vi "SetPersistentConfiguration.vi"(8 "ErrorIn":errorcluster, 9 "DataIn":variant, 11 "ReferenceIn":refnum<class "DemoApplication.lvclass">) -> (0 "ErrorOut":errorcluster, 1 "DataOut":variant, 3 "ReferenceOut":refnum<class "DemoApplication.lvclass">)   [LabVIEW 2021, in "DemoApplication.lvclass"]
uses:
  DemoApplication.lvclass
  C:/Localdata/Projects/TriekselSoft/TriekselsoftApplicationFramework/Source/.Externals/Library_TAF_ApplicationFramework/MasterGUI/MasterGUI.lvclass
  .Externals/Library_TAF_ApplicationFramework/MasterGUI/MasterGUI_MessageData.ctl
  a2d9dd7e-4f73-47a2-b010-087cab1955c7.vi
  7e5dec9a-bf4d-41f7-98bf-8bf962ae9346.vi
  <vilib>/Utility/LVClass/Get LV Class Name.vi
  .Externals/Library_TAF_ApplicationFramework/MasterGUI/MainGUIRepository.vi
  .Externals/Library_TAF_ApplicationFramework/MasterGUI/MasterGUI.lvclass
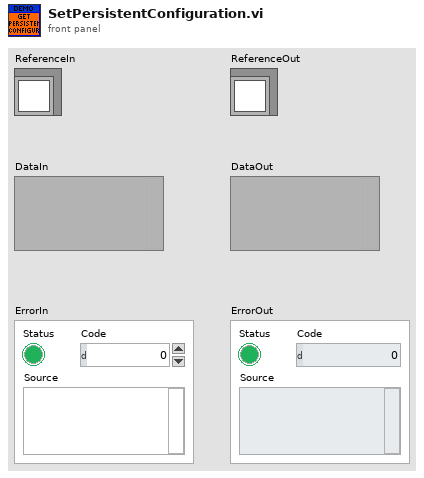
[diagram p1: front panel]
types:
  T1 = typedef "MasterGUI.lvclass/MasterGUI_MessageData.ctl" = cluster{"ShowWindow":cluster{"Send":cluster{"Show":bool}, "Receive":cluster{"Dummy":bool}}}
  T2 = typedef "DemoApplication.lvclass/ObjectAttributes.ctl" = cluster{"Interfaces":cluster{"Authorizer":refnum<class "IAuthorization.lvclass">, "TextViewer":refnum<class "ITAFTextViewer.lvclass">, "ApplicationConfiguration":refnum<class "IApplicationConfiguration.lvclass">, "Tracer":refnum<class "IFrontPanel.lvclass">}, "Persistent":cluster{"MenuEnables":cluster{"MenuTag":string, "MenuExpression":string}[], "TextDockSubPanelName":string}}
  T3 = cluster{"MenuEnables":cluster{"MenuTag":string, "MenuExpression":string}[], "TextDockSubPanelName":string}
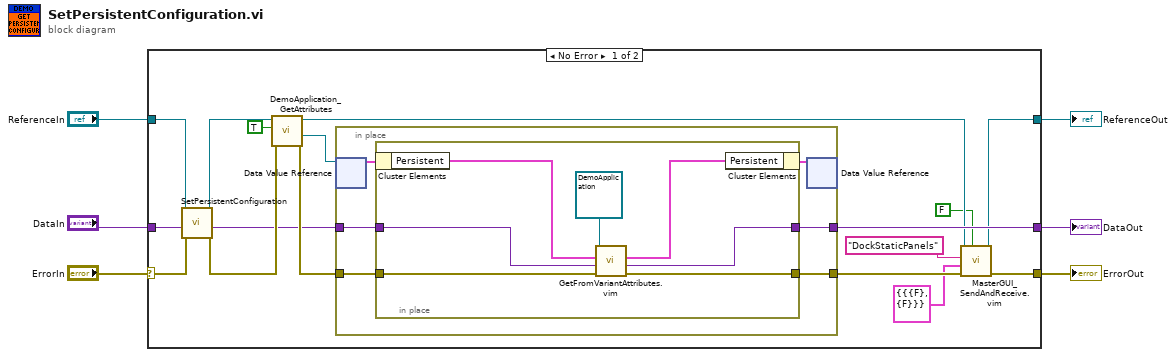
[diagram p0: block diagram]
diagram:
  n1 = case shown="No Error" "ErrorIn" {
    selector: "ErrorIn" -> [w22 w39]
    tunnel: [w19 w39] -> w5
    tunnel: [w10 w38] -> w3
    tunnel: "ReferenceIn" -> [w12 w38]
    tunnel: [w18 w37] -> w2
    tunnel: "DataIn" -> [w14 w37]
    frame No Error {
      n2 = call-parent "SetPersistentConfiguration.vi"("ErrorIn"=w22, "DataIn"=w14, "ReferenceIn"=w12) -> ("ErrorOut"=w21:errorcluster, "DataOut"=w15:variant, "ReferenceOut"=w13:refnum<class "DemoApplication.lvclass">)  [unwired: 6 in]
      n3 = call "DemoApplication_GetAttributes.vi"("ErrorIn"=w21, "OnlyGetDvrReference(False)"=TRUE, "ReferenceIn"=w13) -> ("ErrorOut"=w23:errorcluster, "DataRef"=w16:refnum<data-value>, "ReferenceOut"=w11:refnum<class "DemoApplication.lvclass">)  [unwired: 5 in, 1 out]
      n4 = in-place {
        in-place-border: w23 -> [w29]
        in-place-border: [w28] -> w20
        in-place-border: w15 -> [w27]
        in-place-border: [w26] -> w18
        n5 = in-place-dvr #1(w16) -> (w25:T2)  [unwired: 1 out]
        n6 = in-place {
          in-place-border: w29 -> [w36]
          in-place-border: [w35] -> w28
          in-place-border: w27 -> [w34]
          in-place-border: [w33] -> w26
          n7 = in-place-cluster #2(w25) -> ("Persistent"=w31:T3)
          n8 = call "GetFromVariantAttributes.vim"("ErrorIn"=w36, "DataInIn"=w34, "PersistentDataType"=w31, "Object"=refnum<class "DemoApplication.lvclass"> refnum ("VerticalButtonBar")) -> ("ErrorOut"=w35:errorcluster, "DataOut"=w33:variant, "PersistentDataOut"=w30:T3)  [unwired: 5 in]
          n9 = in-place-cluster #2("Persistent"=w30) -> (w24:T2)
        }
        n10 = in-place-dvr #1(w24) -> ()  [unwired: 2 out]
      }
      n11 = call "MasterGUI_SendAndReceive.vim"("ShouldWeWaitForResponse"=FALSE, "ErrorIn"=w20, "Data"=T1 {"ShowWindow"={"Send"={"Show"=FALSE}, "Receive"={"Dummy"=FALSE}}} ("MessageData"), "Command"="DockStaticPanels", "ReferenceIn"=w11) -> ("ErrorOut"=w19:errorcluster, "ReferenceOut"=w10:refnum<class "DemoApplication.lvclass">)  [unwired: 4 in, 1 out]
    }
    frame Error {
    }
  }
  "ErrorOut" <- w5
  "ReferenceOut" <- w3
  "DataOut" <- w2
